vi "Decript UDP Message.vi"(8 "Error In":errorcluster, 10 "UDP Message":u8[](array[numeric])) -> (0 "Error Out":errorcluster, 1 "Memory":dbl[](array[numeric]), 2 "Analog Input":dbl[](array[numeric]), 3 "Digital Input":bool[](array[boolean]), 4 "CPU":u32[](array[numeric]))   [LabVIEW 2021, in "Main HMI.lvlib"]
uses:
  Main HMI.lvlib
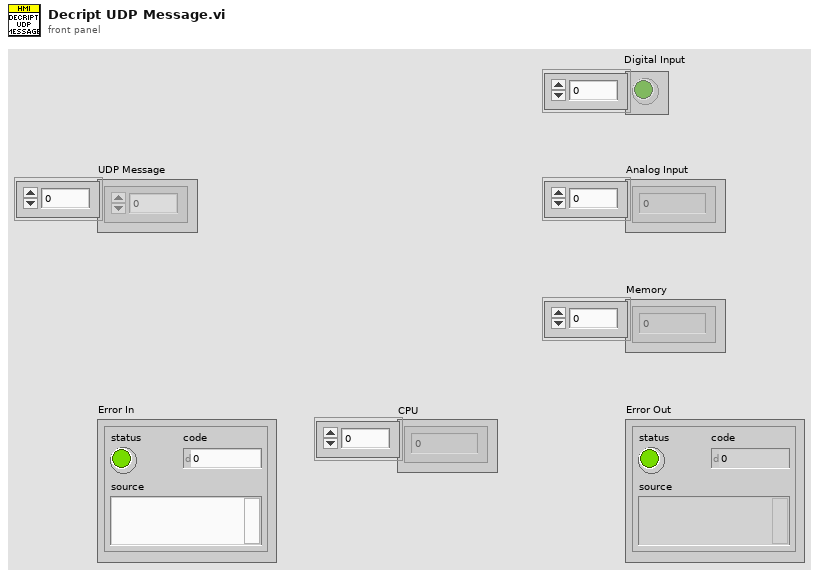
[diagram p1: front panel]
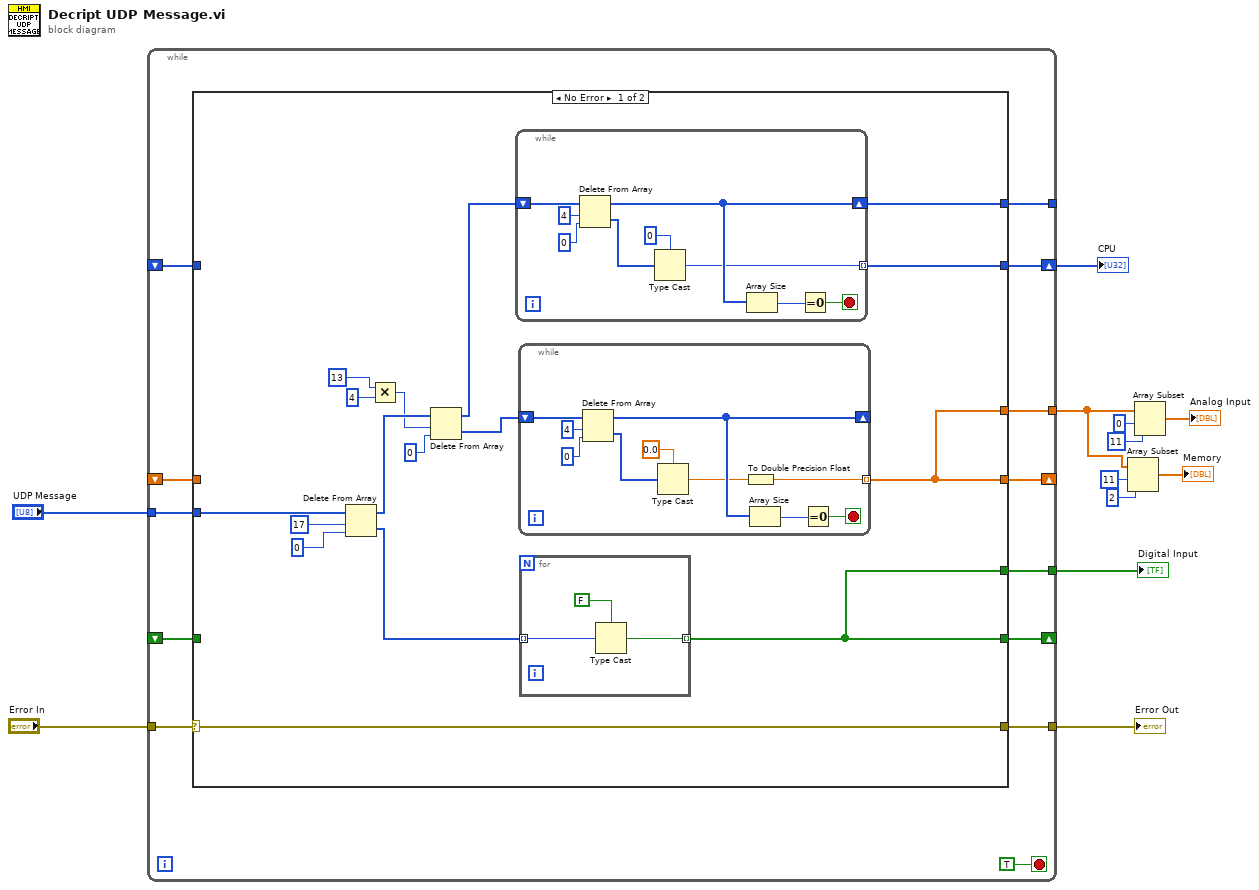
[diagram p0: block diagram]
diagram:
  n1 = while {
    tunnel: "UDP Message" -> [w25]
    tunnel: [w24] -> w11
    tunnel: [w23] -> w2
    tunnel: "Error In" -> [w21]
    tunnel: [w20] -> w9
    shift-right: [w19] -> _
    shift-left: _ -> [w18]
    shift-right: [w17] -> _
    shift-left: _ -> [w16]
    tunnel: [w15] -> _
    shift-right: [w14] -> w1
    shift-left: _ -> [w13]
    stop <- TRUE stop-if-true
    n2 = case shown="No Error" w21 {
      selector: w21 -> [w37 w65]
      tunnel: w25 -> [w39 _]
      tunnel: [w36 w66] -> w24
      tunnel: [w35 w67] -> w23
      tunnel: [w37 w65] -> w20
      tunnel: [w36 w66] -> w19
      tunnel: w18 -> [_ w66]
      tunnel: [w35 w67] -> w17
      tunnel: w16 -> [_ w67]
      tunnel: [w27 w64] -> w15
      tunnel: [w26 w64] -> w14
      tunnel: w13 -> [_ w64]
      frame No Error {
        n3 = Delete From Array(array=w39, length=17, index=0) -> (deleted portion=w38:u8[], array with subset deleted=w34:u8[])
        n4 = Multiply(x=13 ("length"), y=4) -> (x*y=w30:i32)
        n5 = Delete From Array(array=w34, length=w30, index=0) -> (deleted portion=w33:u8[], array with subset deleted=w28:u8[])
        n6 = while {
          shift-right: [w43] -> w27
          shift-left: w28 -> [w50]
          tunnel: [w42] -> w26 mode=indexing
          stop <- w45 stop-if-true
          n7 = Delete From Array(array=w50, length=4, index=0) -> (deleted portion=w47:u8[], array with subset deleted=w43:u8[])
          n8 = Type Cast(type=u32 0, x=w47) -> (*(type *) &x=w42:u32)
          n9 = Array Size(array=w43) -> (size(s)=w44:i32)
          n10 = Equal To 0?(x=w44) -> (x = 0?=w45:bool)
        }
        n11 = while {
          shift-right: [w53] -> _
          shift-left: w33 -> [w60]
          tunnel: [w51] -> w35 mode=indexing
          stop <- w55 stop-if-true
          n12 = Delete From Array(array=w60, length=4, index=0) -> (deleted portion=w57:u8[], array with subset deleted=w53:u8[])
          n13 = Type Cast(type=sgl 0.0, x=w57) -> (*(type *) &x=w52:sgl)
          n14 = To Double Precision Float(number=w52) -> (double precision float=w51:dbl)
          n15 = Array Size(array=w53) -> (size(s)=w54:i32)
          n16 = Equal To 0?(x=w54) -> (x = 0?=w55:bool)
        }
        n17 = for {
          tunnel: w38 -> [w63] mode=indexing
          tunnel: [w61] -> w36 mode=indexing
          n18 = Type Cast(type=FALSE, x=w63) -> (*(type *) &x=w61:bool)
        }
      }
      frame Error {
      }
    }
  }
  "Error Out" <- w9
  "Digital Input" <- w11
  "CPU" <- w1
  n19 = Array Subset(array=w2, index=11, length=2) -> (→"Memory":dbl[])
  n20 = Array Subset(array=w2, index=0, length=11) -> (→"Analog Input":dbl[])
